vi "genRandStreamOdor.vi"(8 "error in (no error)":errorcluster, 11 "Odor in":refnum<class "Odor.lvclass">) -> (0 "error out":errorcluster, 3 "Odor out":refnum<class "Odor.lvclass">)   [LabVIEW 2014, in "Odor.lvclass"]
uses:
  Odor.lvclass
  Odor.lvclass/Odor.ctl
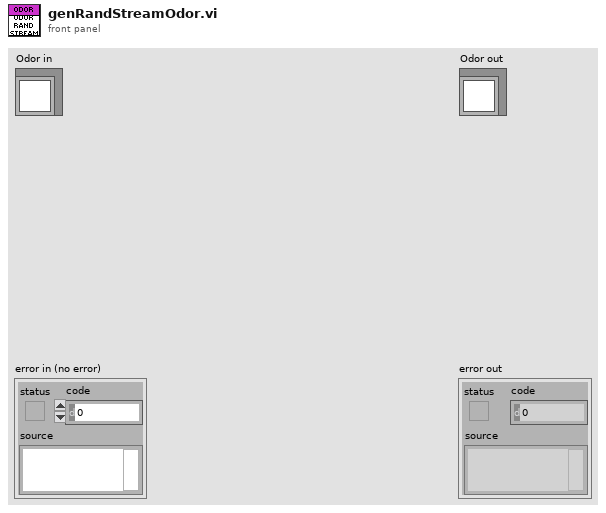
[diagram p1: front panel]
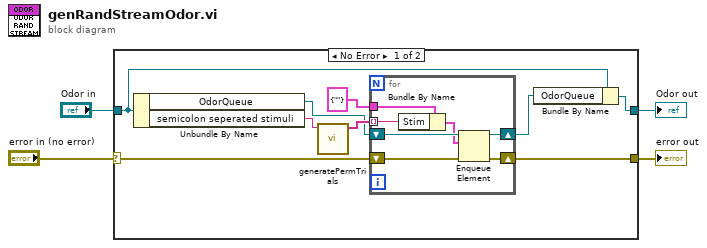
[diagram p0: block diagram]
diagram:
  n1 = case shown="No Error" "error in (no error)" {
    selector: "error in (no error)" -> [w11 w22]
    tunnel: [w10 w22] -> w3
    tunnel: [w7 w21] -> w1
    tunnel: "Odor in" -> [w8 w21]
    frame No Error {
      n2 = Unbundle By Name(w8) -> ("OdorQueue"=w9:refnum<queue>, "semicolon seperated stimuli"=w5:string)
      n3 = call "generatePermTrials.vi"("semicolon seperated stimuli"=w5) -> ("perfmutated trials"=w12:string[])  [unwired: 9 in, 1 out]
      n4 = for {
        shift-right: [w19] -> w10
        shift-left: w11 -> [w20]
        shift-right: [w17] -> w6
        shift-left: w9 -> [w18]
        tunnel: cluster{"Stim":string} {"Stim"=""} ("Stim element") -> [w16]
        tunnel: w12 -> [w15] mode=indexing
        n5 = Bundle By Name(cluster=w16, "Stim"=w15) -> (w14:cluster{"Stim":string})
        n6 = Enqueue Element(queue=w18, element=w14, error in (no error)=w20) -> (queue out=w17:refnum<queue>, error out=w19:errorcluster)  [unwired: 1 in, 1 out]
      }
      n7 = Bundle By Name(cluster=w8, "OdorQueue"=w6) -> (w7:refnum<class "Odor.lvclass">)
    }
    frame Error {
    }
  }
  "error out" <- w3
  "Odor out" <- w1
